vi "AddNeighbour.vi"(8 "Error In":errorcluster, 10 "Neighbour":refnum<class "12_Cave.lvclass">, 11 "reference in":refnum<class "12_Cave.lvclass">) -> (0 "Error Out":errorcluster, 3 "reference out":refnum<class "12_Cave.lvclass">)   [LabVIEW 2020, in "12_Cave.lvclass"]
uses:
  12_Cave.lvclass
  325e48ee-9957-4f45-a651-97560f8b1902.vi
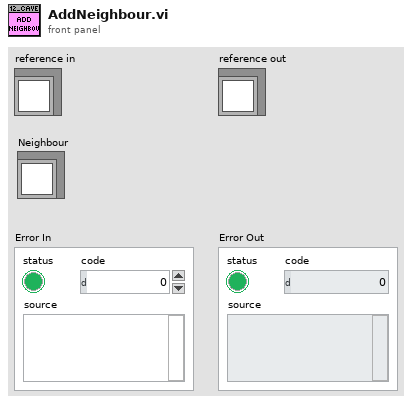
[diagram p1: front panel]
types:
  T1 = typedef "12_Cave.lvclass/ObjectAttributes.ctl" = cluster{"Neighbours":refnum<class "12_Cave.lvclass">[], "Is Big":bool, "Name":string}
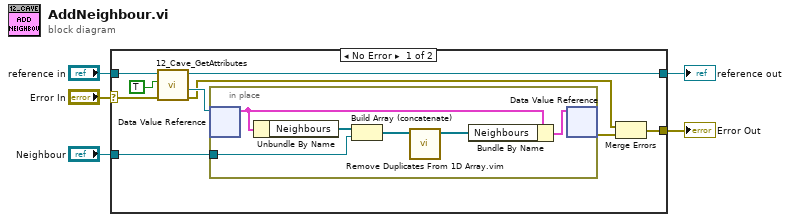
[diagram p0: block diagram]
diagram:
  n1 = case shown="No Error" "Error In" {
    selector: "Error In" -> [w12 w22]
    tunnel: [w7 w22] -> w4
    tunnel: [w13 w21] -> w2
    tunnel: "reference in" -> [w14 w21]
    tunnel: "Neighbour" -> [w6 _]
    frame No Error {
      n2 = call "12_Cave_GetAttributes.vi"("error in (no error)"=w12, "OnlyGetDvrReference(False)"=TRUE, "reference in"=w14) -> ("error out"=w8:errorcluster, "DataRef"=w9:refnum<data-value>, "reference out"=w13:refnum<class "12_Cave.lvclass">)  [unwired: 5 in, 1 out]
      n3 = in-place {
        in-place-border: w6 -> [w17]
        n4 = in-place-dvr #1(w9) -> (w19:T1)  [unwired: 1 out]
        n5 = Unbundle By Name(w19) -> ("Neighbours"=w18:refnum<class "12_Cave.lvclass">[])
        n6 = Build Array (concatenate)(w18, w17) -> (w16:refnum<class "12_Cave.lvclass">[])
        n7 = call "Remove Duplicates From 1D Array.vim"("array"=w16) -> ("array with duplicates removed"=w15:refnum<class "12_Cave.lvclass">[])  [unwired: 10 in]
        n8 = Bundle By Name(cluster=w19, "Neighbours"=w15) -> (w20:T1)
        n9 = in-place-dvr #1(w20) -> (w10:errorcluster)  [unwired: 1 out]
      }
      n10 = Merge Errors(w8, w10) -> (w7:errorcluster)
    }
    frame Error {
    }
  }
  "Error Out" <- w4
  "reference out" <- w2
